vi "TestVI.vi"() -> ()   [LabVIEW 2012]
panel:
  in  "working directory":path=path "C:/perlTest"
  in  "command line":string="perl MyScript.pl argument1"
  out "error out":errorcluster
  out "standard error":string
  out "standard output":string
  # "This command will run this in a new process"
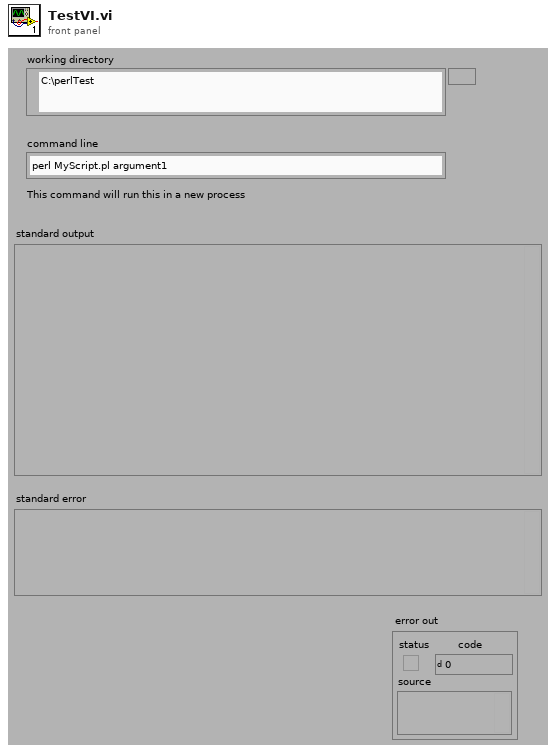
[diagram p1: front panel]
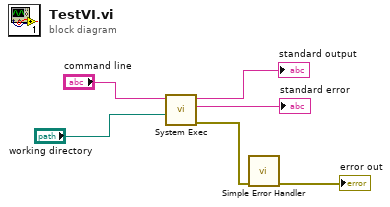
[diagram p0: block diagram]
diagram:
  n1 = call <vilib>:"System Exec.vi"("working directory"="working directory", "command line"="command line") -> ("error out"=w2:errorcluster, "standard error"=→"standard error":string, "standard output"=→"standard output":string)  [unwired: 4 in, 3 out]
  n2 = call <vilib>:"Simple Error Handler.vi"("error in (no error)"=w2) -> ("error out"=→"error out":errorcluster)  [unwired: 1 in, 7 out]
